vi "Condition Type.vi"(11 "HighLimit Condition Config in":refnum<class "HighLimit Condition Config.lvclass">) -> (2 "Condition Type":string)   [LabVIEW 2020, in "VolatusSeqConfig.lvlib" / "HighLimit Condition Config.lvclass"]
uses:
  HighLimit Condition Config.lvclass
  HighLimit Condition Config.lvclass/HighLimit Condition Config.ctl
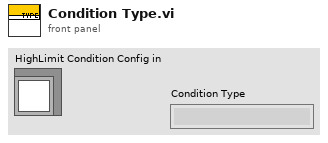
[diagram p1: front panel]
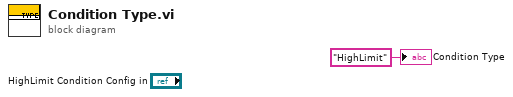
[diagram p0: block diagram]
diagram:
  "Condition Type" <- "HighLimit" ("Condition Type")
